vi "Build Perfect Strips Image.vi"(8 "error in (no error)":errorcluster, 11 "Angle (degrees)":sgl format="%.2f") -> (0 "error out":errorcluster, 3 "Image Out":T1)   [LabVIEW 2016]
uses:
  <vilib>/vision/Image Controls.llb/IMAQ Image.ctl
  <vilib>/vision/NI_Vision_Development_Module.lvlib
panel:
  out "Strips":T1(plugin-control)
  in  "File Path":path=path "D:/Documents/School/Brookhaven/Images/Pixel to Micron Test/image_000_600_60_15.png"
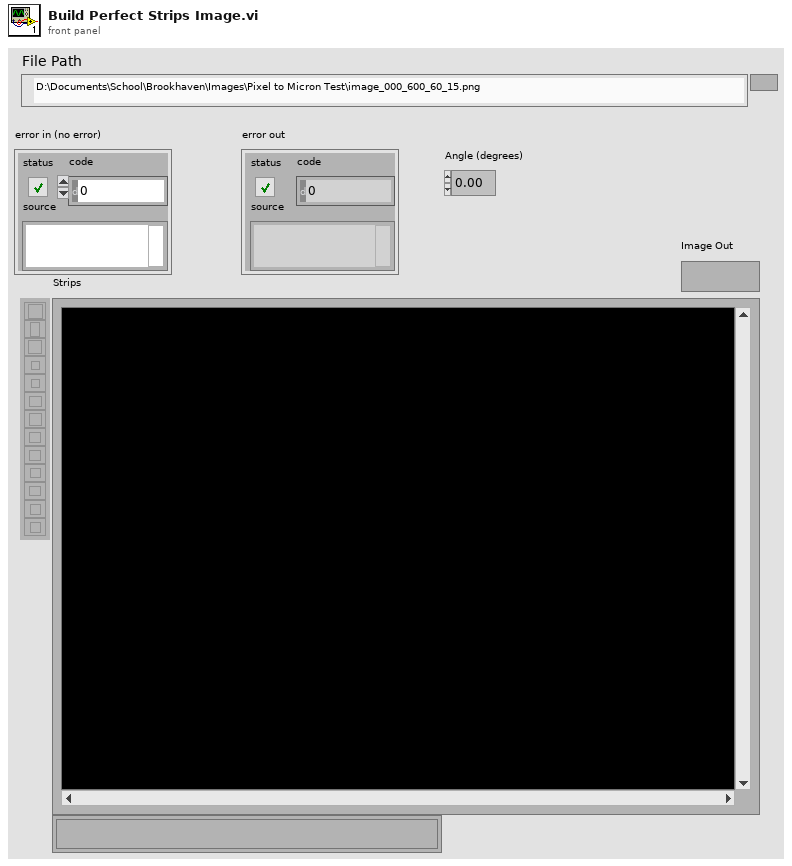
[diagram p1: front panel]
types:
  T1 = typedef "IMAQ Image.ctl" = refnum<image>
  T2 = typedef "Image Type" = u32
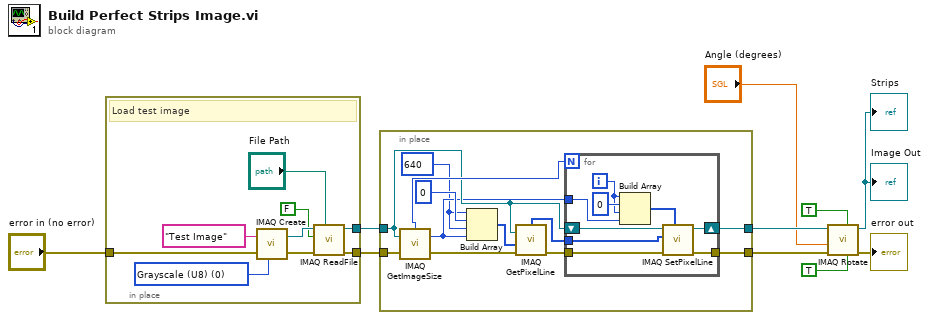
[diagram p0: block diagram]
diagram:
  n1 = in-place {
    in-place-border: [w11] -> w9
    in-place-border: [w13] -> w8
    in-place-border: "error in (no error)" -> [w12]
    w16 = T2 0 items=["Grayscale (U8)", "Grayscale (I16)", "Grayscale (SGL)", "Complex (CSG)", "RGB (U32)", "HSL (U32)", "RGB (U64)", "Grayscale (U16)"] ("Image Type")
    # "Load test image"
    n2 = call "IMAQ Create"("Image Name"="Test Image", "Image Type"=w16, "error in (no error)"=w12) -> ("New Image"=w17:T1, "error out"=w14:errorcluster)  [unwired: 2 in]
    n3 = call "IMAQ ReadFile"("File Path"="File Path", "error in (no error)"=w14, "Load Color Palette? (No)"=FALSE, "Image"=w17) -> ("error out"=w13:errorcluster, "Image Out"=w11:T1)  [unwired: 3 in, 3 out]
  }
  n4 = in-place {
    in-place-border: w9 -> [w29]
    in-place-border: [w24] -> w7
    in-place-border: w8 -> [w23]
    in-place-border: [w20] -> w3
    w25 = 640
    n5 = call "IMAQ GetImageSize"("Image"=w29, "error in (no error)"=w23) -> ("Y Resolution"=w27:i32, "X Resolution"=w31:i32, "error out"=w22:errorcluster)  [unwired: 2 in]
    n6 = Build Array(w25, 0, w25, w27) -> (w26:i32[])
    n7 = call "IMAQ GetPixelLine"("error in (no error)"=w22, "Line Coordinates"=w26, "Image"=w29) -> ("error out"=w21:errorcluster, "Pixels Line (U8)"=w30:u8[])  [unwired: 1 in, 3 out]
    n8 = for {
      N: w31 -> [_]
      tunnel: w30 -> [w39]
      shift-right: [w38] -> w24
      shift-left: w29 -> [w40]
      tunnel: w27 -> [w35]
      tunnel: w21 -> [w33]
      tunnel: [w32] -> w20
      i -> [w36]
      n9 = Build Array(w36, 0, w36, w35) -> (w34:i32[])
      n10 = call "IMAQ SetPixelLine"("Line Coordinates"=w34, "error in (no error)"=w33, "Pixels Line (U8)"=w39, "Image"=w40) -> ("error out"=w32:errorcluster, "Image Out"=w38:T1)  [unwired: 6 in]
    }
  }
  n11 = call "IMAQ Rotate"("Use Bilinear Interpolation"=TRUE, "Maintain Size"=TRUE, "error in (no error)"=w3, "Angle (degrees)"="Angle (degrees)", "Image Src"=w7) -> ("error out"=→"error out":errorcluster, "Image Dst Out"=→"Strips" →"Image Out":T1)  [unwired: 5 in]
